vi "ThreeButtonDialogWithTimeout.vi"(4 "Allow user to close window? (TRUE)":bool=TRUE, 5 "Timeout (s)":dbl=15.0 caption="Time Target (s)", 6 "Keyboard Shortcuts (Left is <Enter>)":T1={"Left Button Key Shortcut"={"Control"=FALSE, "Shift"=FALSE, "Key"="<Enter>"}, "Center Button Key Shortcut"={"Control"=FALSE, "Shift"=FALSE, "Key"=""}, "Right Button Key Shortcut"={"Control"=FALSE, "Shift"=FALSE, "Key"=""}}, 7 "Window Title (\"\")":string, 8 "Right Button Text (\"Cancel\")":string="Cancel", 9 "Center Button Text (\"No\")":string="No", 10 "Default Button Text (\"Yes\")":string="Yes", 11 "message":string) -> (2 "Which Button?":T2(ring))   [LabVIEW 2016]
doc: "Displays a dialog box that contains a message and a single \"OK\" button using the One Button Dialog VI. This VI will automatically press \"OK\" after Timeout (s) has occured."
uses:
  user32.dll
panel:
  in  "Stopped":bool
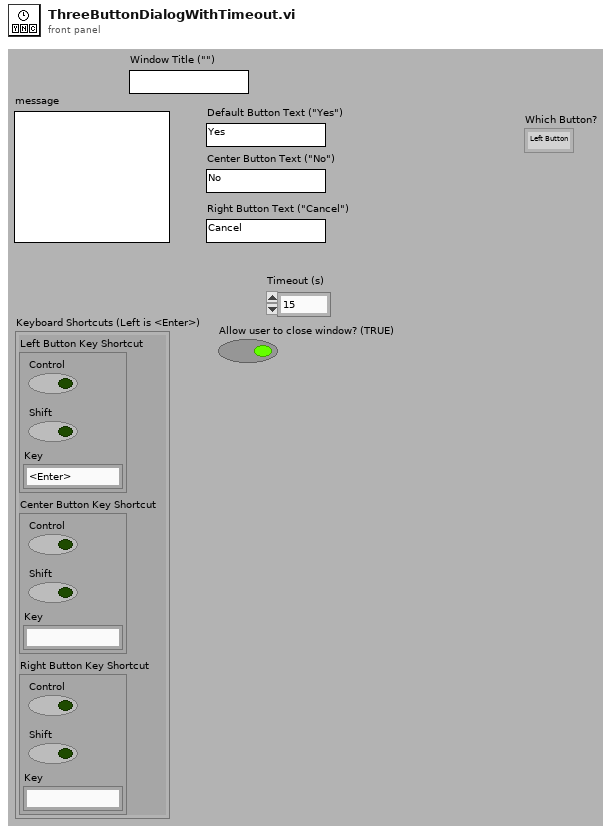
[diagram p1: front panel]
types:
  T1 = cluster{"Left Button Key Shortcut":cluster{"Control":bool, "Shift":bool, "Key":string}, "Center Button Key Shortcut":cluster{"Control":bool, "Shift":bool, "Key":string}, "Right Button Key Shortcut":cluster{"Control":bool, "Shift":bool, "Key":string}}
  T2 = enum16{"Left Button", "Center Button", "Right Button", "Window Close"}
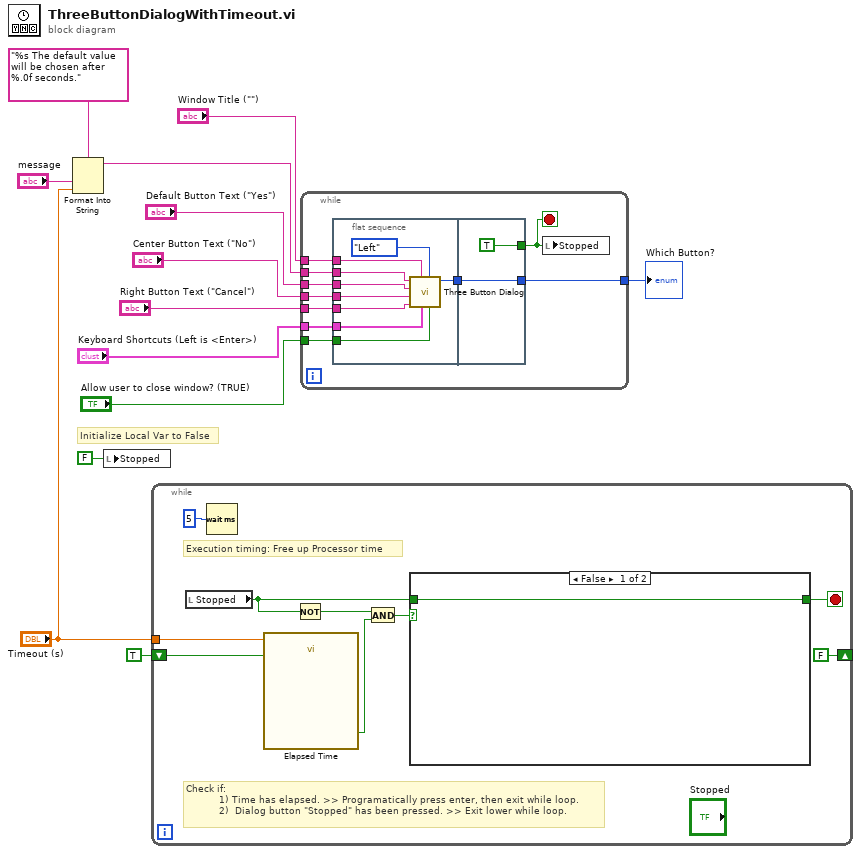
[diagram p0: block diagram]
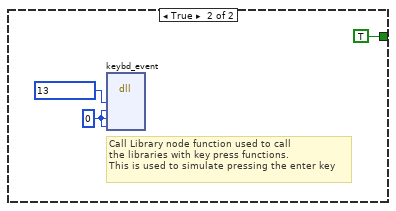
[diagram p2: hidden frame]
diagram:
  # "Initialize Local Var to False"
  n1 = Format Into String(format string="%s The default value will be chosen after %.0f seconds.", "message", "Timeout (s)") -> (resulting string=w2:string)  [unwired: 2 in, 1 out]
  n2 = local write "Stopped"(FALSE ("Stopped")) -> ()
  n3 = while {
    tunnel: "Timeout (s)" -> [w16]
    shift-right: [FALSE ("Stopped")] -> _
    shift-left: TRUE ("Stopped") -> [w15]
    stop <- w22 stop-if-true
    # "Check if:\n           1) Time has elapsed. >> Programatically press enter, then exit while loop.\n           2)  Dialog button \"Stopped\" has been pressed. >> Exit lower while loop."
    # "Execution timing: Free up Processor time"
    n4 = local read "Stopped"() -> (w18:bool)
    n5 = Wait (ms)(milliseconds to wait=u32 5) -> ()  [unwired: 1 out]
    n6 = call "Elapsed Time"("Time Target (s)"=w16, "Reset"=w15) -> ("Time has Elapsed"=w19:bool)  [unwired: 10 in, 7 out]
    n7 = Not(x=w18) -> (.not. x?=w20:bool)
    n8 = And(x=w20, y=w19) -> (x .and. y?=w21:bool)
    n9 = case shown="False" w21 {
      tunnel: [w23 TRUE] -> w22
      tunnel: w18 -> [w23 _]
      frame False {
      }
      frame True {
        w25 = u8 0 ("bScan")
        # "Call Library node function used to call \nthe libraries with key press functions. \nThis is used to simulate pressing the enter key"
        n10 = dll-call lib="user32.dll" fn="keybd_event"("bVk"=u8 13 ("Virtual Key"), "bScan"=w25, "dwFlags"=w25, "dwExtraInfo"=w25) -> ()  [unwired: 8 in, 2 out]
      }
    }
  }
  n11 = while {
    tunnel: [w34] -> w12
    tunnel: "Window Title (\"\")" -> [w33]
    tunnel: w2 -> [w32]
    tunnel: "Default Button Text (\"Yes\")" -> [w31]
    tunnel: "Center Button Text (\"No\")" -> [w30]
    tunnel: "Right Button Text (\"Cancel\")" -> [w29]
    tunnel: "Keyboard Shortcuts (Left is <Enter>)" -> [w28]
    tunnel: "Allow user to close window? (TRUE)" -> [w27]
    stop <- w36 stop-if-true
    n12 = flat-sequence {
      tunnel: [w45] -> w35
      tunnel: w33 -> [w44]
      tunnel: w32 -> [w43]
      tunnel: w31 -> [w42]
      tunnel: w30 -> [w41]
      tunnel: w29 -> [w40]
      tunnel: w28 -> [w39]
      tunnel: w27 -> [w38]
      tunnel: [TRUE] -> w36
      tunnel: w35 -> [w46]
      tunnel: [w46] -> w34
      frame #0 {
        n13 = call <vilib>:"Three Button Dialog.vi"("Allow user to close window? (TRUE)"=w38, "Justify Message (Left)"=enum16{"Left", "Center", "Right"}."Left", "Keyboard Shortcuts (Left is <Enter>)"=w39, "Window Title (\"\")"=w44, "Right Button Text (\"Cancel\")"=w40, "Center Button Text (\"No\")"=w41, "Left Button Text (\"Yes\")"=w42, "message"=w43) -> ("Which Button?"=w45:T2)  [unwired: 3 in]
      }
      frame #1 {
      }
    }
    n14 = local write "Stopped"(w36) -> ()
  }
  "Which Button?" <- w12
